vi "FXP_diag_state_space.vi"() -> ()   [LabVIEW 2017]
uses:
  <vilib>/Platform/TimedLoop/XDataNode/timing_clust.ctl
  <vilib>/Platform/TimedLoop/XDataNode/nitl_modes.ctl
  <vilib>/Platform/TimedLoop/XDataNode/wakeup.ctl
  <vilib>/rvi/IPIntegrationNode/IPINode_Typedef/niFpgaIPINodeSupportedFamilies.ctl
  <vilib>/rvi/Emulation/niFpgaSctlEmulationGetInTimedLoop.vi
  <vilib>/rvi/Emulation/niFpgaEmulationReportErrorSimple.vi
  <vilib>/rvi/Emulation/niFpgaGetClockAttributes.vi
  <vilib>/rvi/Emulation/niFpgaCriticalErrorInLSC.vi
  <vilib>/rvi/Memory/Memory_Emulation/nirvimemoryFastEmulation.vi
  <vilib>/rvi/Memory/Memory_Emulation/nirvimemoryEmulation.vi
  <vilib>/rvi/Emulation/niFpgaEmulationIsFPGAContextNoSignature.vi
  <vilib>/rvi/DataTransferAndStorage/Container/Common/niFpgaContainerGetUniqueNameForEmu.vi
  <vilib>/rvi/Emulation/niFpgaProcessEmulError.vi
  <vilib>/rvi/errors/nirviReportUnexpectedCaseInternalError (U32).vi
  <vilib>/rvi/IPIntegrationNode/IPINode_Utilities/niFpgaIPINodeSimCore.vi
  <vilib>/Platform/TimedLoop/XDataNode/XDataNode.xnode
  <vilib>/rvi/DataTransferAndStorage/Container/XNode/niFpgaContainer.xnode
  <vilib>/rvi/XilinxIP/XIPIN_XNode/niFpgaXIPIN.xnode
  FXP_diag_state_space/Multiply Accumulator/Multiply_Accumulator_9748E7119E544630B9E04781A333D267.dll
  <vilib>/rvi/IPIntegrationNode/IPINode_Xnode/niFpgaIPINode.xnode
  <vilib>/rvi/FXPMathLib/FxpMul/XNode/nifxpmath_Multiplier.xnode
  <vilib>/rvi/FXPMathLib/FxpAdd/XNode/nifxpmath_Add.xnode
  <vilib>/Platform/TimedLoop/XDataNode/XDNodeRunTimeDep.lvlib
  <vilib>/rvi/FXPMathLib/sim/FxpSim.dll
panel:
  out "y(k)":fxp<+/-,64,8> format="%.59g"
  in  "Drift_order":u8
  in  "D":fxp<+/-,16,1> format="%.16g"
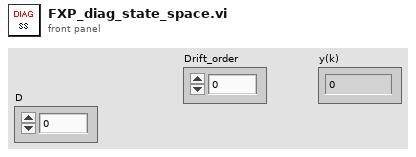
[diagram p1: front panel]
types:
  T1 = typedef "XDNodeRunTimeDep.lvlib/timing_clust.ctl" = cluster{"Expected End [f-1]":u64, "Actual End [f-1]":u64, "Finished Late? [f-1]":bool, "Expected End [i-1]":u64, "Actual End [i-1]":u64, "Finished Late? [i-1]":bool, "Expected Start [i]":u64, "Actual Start [i]":u64, "Expected Start [f]":u64, "Actual Start [f]":u64, "Source Name":string, "Structure Name":string, "Period":i64, "Deadline":i64, "Offset":i64, "Start":i64, "Priority":i32, "Timeout":i32, "Mode":T2, "Wakeup Reason":T3, "Error":errorcluster, "Source Type":string, "Secondary Source Type":string, "Global End Time":u64, "Global Start Time":u64, "Frame Duration":u64, "Iteration Duration":u64, "Assigned CPU":i32, "I/O Scan Engine Mode":u32}
  T2 = typedef "XDNodeRunTimeDep.lvlib/nitl_modes.ctl" = enum32{"No Change", "Process missed periods, maintain original phase", "Discard missed periods, maintain original phase", "Process missed periods, ignore original phase", "Discard missed periods, ignore original phase"}
  T3 = typedef "XDNodeRunTimeDep.lvlib/wakeup.ctl" = enum32{"Normal", "Aborted", "Asynchronous wakeup", "Timing source error", "Timed loop error", "Timeout"}
  T4 = typedef "niFpgaIPINodeSupportedFamilies.ctl" = cluster{"unlimited?":bool, "supported targets":string[]}
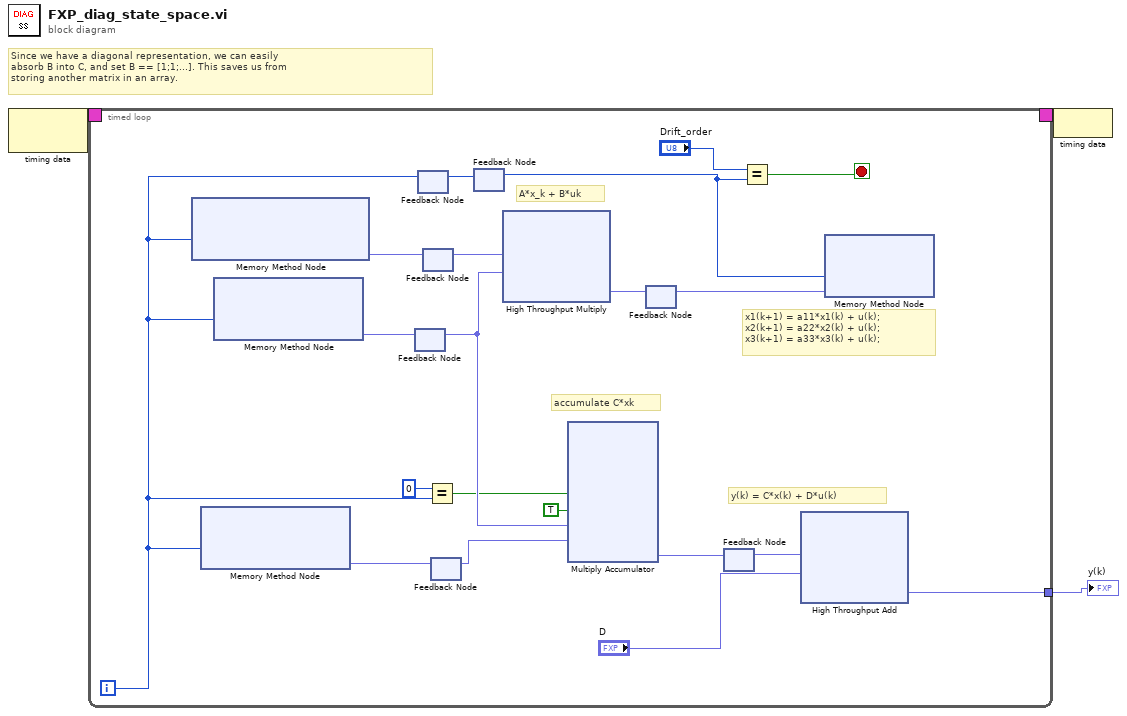
[diagram p0: block diagram]
diagram:
  # "Since we have a diagonal representation, we can easily\nabsorb B into C, and set B == [1;1;...]. This saves us from \nstoring another matrix in an array."
  n1 = node-c288() -> (w3:T1)  [unwired: 1 in]
  n2 = timed-loop {
    timing: w3 -> [_]
    timing-out: [_] -> w2
    tunnel: [w4] -> w1
    i -> [w7]
    stop <- w10 stop-if-true
    # "accumulate C*xk"
    # "A*x_k + B*uk"
    # "x1(k+1) = a11*x1(k) + u(k);\nx2(k+1) = a22*x2(k) + u(k);\nx3(k+1) = a33*x3(k) + u(k);"
    # "y(k) = C*x(k) + D*u(k)"
    n3 = xnode ("Memory Method Node")("Address"=w7) -> ("Data"=w23:fxp<+/-,32,1>)  [unwired: 1 in, 1 out]
    n4 = xnode ("Memory Method Node")("Address"=w7) -> ("Data"=w16:fxp<+/-,32,1>)  [unwired: 1 in, 1 out]
    n5 = xnode ("Memory Method Node")("Address"=w7) -> ("Data"=w21:fxp<+/-,32,6>)  [unwired: 1 in, 1 out]
    n6 = feedback #1() -> (w17:fxp<+/-,32,6>)  [unwired: 1 in]
    n7 = feedback-in #1(w21) -> ()
    n8 = feedback #2() -> (w20:i32)  [unwired: 1 in]
    n9 = feedback-in #2(w7) -> ()
    n10 = feedback-in #3(w23) -> ()
    n11 = feedback #3() -> (w22:fxp<+/-,32,1>)  [unwired: 1 in]
    n12 = Equal?(x=0, y=w7) -> (x = y?=w8:bool)
    n13 = feedback #4() -> (w15:fxp<+/-,32,1>)  [unwired: 1 in]
    n14 = feedback-in #4(w16) -> ()
    n15 = feedback #5() -> (w11:i32)  [unwired: 1 in]
    n16 = feedback-in #5(w20) -> ()
    n17 = xnode "High Throughput Multiply"("x"=w22, "y"=w17) -> ("x*y"=w19:fxp<+/-,64,7>)
    n18 = xnode ("Multiply Accumulator")("sclr"=w8, "bypass"=TRUE, "a"=w17, "b"=w15) -> ("s"=w14:fxp<+/-,36,7>)  [unwired: 1 in]
    n19 = feedback #6() -> (w18:fxp<+/-,64,7>)  [unwired: 1 in]
    n20 = feedback-in #6(w19) -> ()
    n21 = feedback #7() -> (w13:fxp<+/-,36,7>)  [unwired: 1 in]
    n22 = feedback-in #7(w14) -> ()
    n23 = Equal?(x="Drift_order", y=w11) -> (x = y?=w10:bool)
    n24 = xnode "High Throughput Add"("x"=w13, "y"="D") -> ("x+y"=w4:fxp<+/-,37,8>)
    n25 = xnode ("Memory Method Node")("Address"=w11, "Data"=w18) -> ()  [unwired: 1 in, 1 out]
  }
  "y(k)" <- w1
  n26 = node-c288(w2) -> ()
